vi "Init.vi"(8 "error in":errorcluster, 10 "Dictionary":refnum<class "Dictionary.lvclass">, 11 "Sorted Object Dictionary in":refnum<class "Sorted Object Dictionary.lvclass">) -> (0 "error out":errorcluster, 3 "Sorted Object Dictionary out":refnum<class "Sorted Object Dictionary.lvclass">)   [LabVIEW 2024, in "Electronic Datasheet.lvlib" / "Sorted Object Dictionary.lvclass"]
doc: "Check if section is not part of infosection\nand if it is an od entry or od subentry"
uses:
  Sorted Object Dictionary.lvclass
  Object Dictionary/Dictionary.lvclass
  Object Dictionary/Dictionary.lvclass/Dictionary.ctl
  Sorted Object Dictionary.lvclass/Sorted Object Dictionary.ctl
  OD Section/Section.lvclass/Section.ctl
  OD Entry/OD Entry.lvclass
  OD Sub-Entry/OD Sub-Entry.lvclass
  OD Section/Section.lvclass
  Electronic Datasheet.lvlib
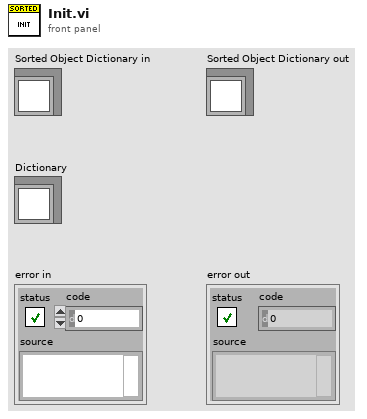
[diagram p1: front panel]
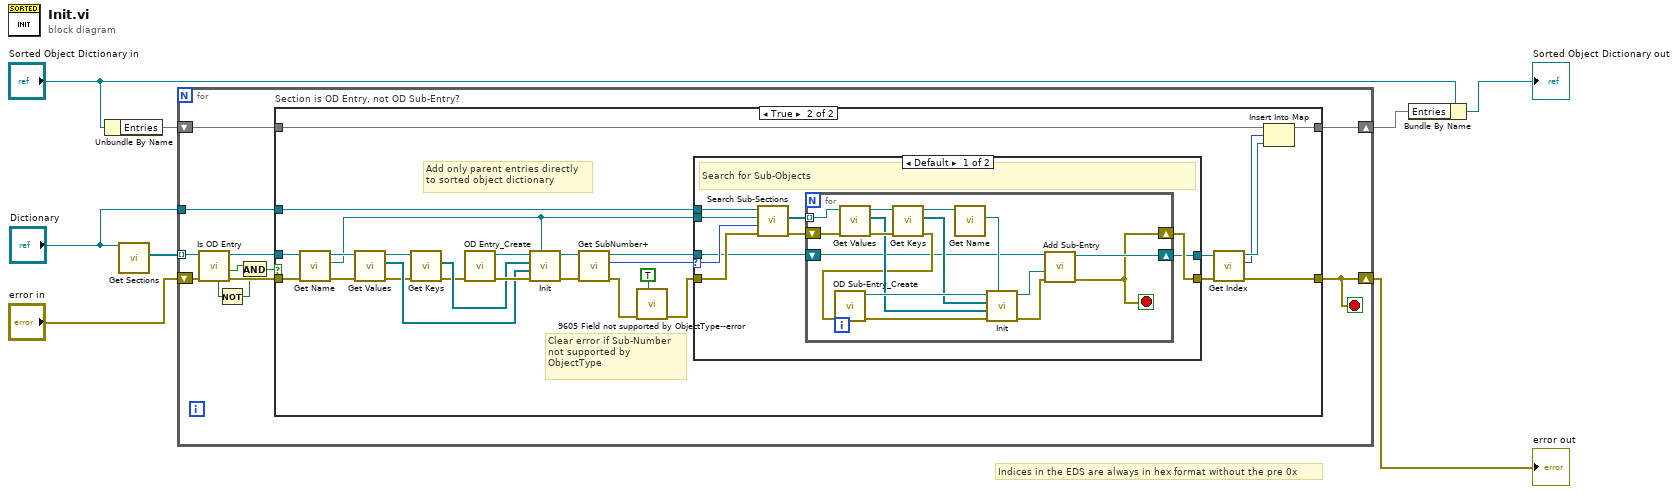
[diagram p0: block diagram]
diagram:
  # "Indices in the EDS are always in hex format without the pre 0x"
  n1 = Unbundle By Name("Sorted Object Dictionary in") -> ("Entries"=w8:map{u16, refnum<class "OD Entry.lvclass">})
  n2 = call "Get Sections.vi"("Dictionary in"="Dictionary") -> ("OD Sections"=w2:refnum<class "Section.lvclass">[])  [unwired: 9 in, 1 out]
  n3 = for {
    tunnel: w2 -> [w16] mode=indexing
    shift-right: [w13] -> w5
    shift-left: w8 -> [w14]
    shift-right: [w15] -> w3
    shift-left: "error in" -> [w18]
    tunnel: "Dictionary" -> [w19]
    stop <- w15 stop-if-true
    n4 = call "Is OD Entry.vi"("error in"=w18, "Section in"=w16) -> ("error out"=w17:errorcluster, "Is OD Entry?"=w11:bool, "Section out"=w20:refnum<class "Section.lvclass">, "Is Sub-Entry?"=w10:bool)  [unwired: 5 in, 1 out]
    n5 = Not(x=w10) -> (.not. x?=w9:bool)
    n6 = And(x=w11, y=w9) -> (x .and. y?=w12:bool)
    n7 = case "Section is OD Entry, not OD Sub-Entry?" shown="True" w12 {
      tunnel: w20 -> [_ w40]
      tunnel: w17 -> [w22 w42]
      tunnel: w19 -> [_ w36]
      tunnel: [w22 w27] -> w15
      tunnel: w14 -> [w21 w29]
      tunnel: [w21 w28] -> w13
      frame False {
      }
      frame True {
        # "Add only parent entries directly\nto sorted object dictionary"
        # "Clear error if Sub-Number\nnot supported by\nObjectType"
        n8 = call "Get Name.vi"("Object Entry in"=w40) -> ("Section Name"=w32:refnum<class "Section Name.lvclass">, "Object Entry out"=w35:refnum<class "Section.lvclass">)  [unwired: 9 in]
        n9 = call "Get Values.vi"("error in (no error)"=w42, "Section in"=w35) -> ("error out"=w43:errorcluster, "Values"=w44:refnum<class "Value.lvclass">[], "Section out"=w46:refnum<class "Section.lvclass">)  [unwired: 7 in]
        n10 = call "Get Keys.vi"("error in"=w43, "Object Entry in"=w46) -> ("error out"=w41:errorcluster, "Keys"=w45:refnum<class "Key Name.lvclass">[])  [unwired: 7 in, 1 out]
        n11 = call "OD Entry_Create.vi"("Error In"=w41) -> ("Error Out"=w48:errorcluster, "reference out"=w47:refnum<class "OD Entry.lvclass">)  [unwired: 9 in]
        n12 = call-dynamic "Init.vi"("Section Name"=w32, "Error In"=w48, "Values"=w44, "Keys"=w45, "reference in"=w47) -> ("Error Out"=w39:errorcluster, "reference out"=w38:refnum<class "OD Entry.lvclass">)  [unwired: 5 in]
        n13 = call "Get SubNumber+.vi"("Error In"=w39, "reference in"=w38) -> ("Error Out"=w34:errorcluster, "SubNumber"=w37:u8, "reference out"=w33:refnum<class "OD Entry.lvclass">)  [unwired: 6 in, 1 out]
        n14 = call "9605 Field not supported by ObjectType--error.vi"("Clear this error?"=TRUE, "error in"=w34) -> ("error out"=w30:errorcluster)  [unwired: 8 in, 1 out]
        n15 = case shown="Default" w37 {
          selector: w37 -> [w54 _]
          tunnel: w36 -> [w57 _]
          tunnel: w30 -> [w55 w75]
          tunnel: w33 -> [w52 w74]
          tunnel: w32 -> [w56 _]
          tunnel: [w50 w75] -> w31
          tunnel: [w49 w74] -> w26
          frame Default {
            # "Search for Sub-Objects"
            n16 = call "Search Sub-Sections.vi"("error in"=w55, "Count"=w54, "Parent Section"=w56, "Dictionary in"=w57) -> ("error out"=w51:errorcluster, "Sub-Sections"=w53:refnum<class "Section.lvclass">[])  [unwired: 4 in, 2 out]
            n17 = for {
              tunnel: w53 -> [w71] mode=indexing
              shift-right: [w58] -> w50
              shift-left: w51 -> [w64]
              shift-right: [w59] -> w49
              shift-left: w52 -> [w62]
              stop <- w58 stop-if-true
              n18 = call "Get Values.vi"("error in (no error)"=w64, "Section in"=w71) -> ("error out"=w68:errorcluster, "Values"=w67:refnum<class "Value.lvclass">[], "Section out"=w69:refnum<class "Section.lvclass">)  [unwired: 7 in]
              n19 = call "Get Keys.vi"("error in"=w68, "Object Entry in"=w69) -> ("error out"=w63:errorcluster, "Keys"=w70:refnum<class "Key Name.lvclass">[], "Object Entry out"=w66:refnum<class "Section.lvclass">)  [unwired: 7 in]
              n20 = call "OD Sub-Entry_Create.vi"("Error In"=w63) -> ("Error Out"=w73:errorcluster, "reference out"=w72:refnum<class "OD Sub-Entry.lvclass">)  [unwired: 9 in]
              n21 = call "Get Name.vi"("Object Entry in"=w66) -> ("Section Name"=w65:refnum<class "Section Name.lvclass">)  [unwired: 9 in, 1 out]
              n22 = call-dynamic "Init.vi"("Section Name"=w65, "Error In"=w73, "Values"=w67, "Keys"=w70, "reference in"=w72) -> ("Error Out"=w60:errorcluster, "reference out"=w61:refnum<class "OD Sub-Entry.lvclass">)  [unwired: 5 in]
              n23 = call "Add Sub-Entry.vi"("Error In"=w60, "OD Sub-Entry"=w61, "reference in"=w62) -> ("Error Out"=w58:errorcluster, "reference out"=w59:refnum<class "OD Entry.lvclass">)  [unwired: 7 in]
            }
          }
          frame 0 {
          }
        }
        n24 = call "Get Index.vi"("Error In"=w31, "reference in"=w26) -> ("Error Out"=w27:errorcluster, "Index"=w24:u16, "reference out"=w25:refnum<class "OD Entry.lvclass">)  [unwired: 7 in]
        n25 = Insert Into Map(map in=w29, key=w24, value=w25) -> (map out=w28:map{u16, refnum<class "OD Entry.lvclass">})  [unwired: 2 out]
      }
    }
  }
  "error out" <- w3
  n26 = Bundle By Name(cluster="Sorted Object Dictionary in", "Entries"=w5) -> (→"Sorted Object Dictionary out":refnum<class "Sorted Object Dictionary.lvclass">)
